vi "setConfiguration.vi"() -> (3 "TCPSettings out":refnum<class "TCPSettings.lvclass">)   [LabVIEW 2016]
uses:
  TCPSettings/TCPSettings.lvclass
  TCPSettings/TCPSettings.lvclass/TCPSettings.ctl
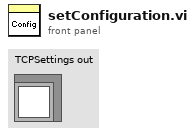
[diagram p1: front panel]
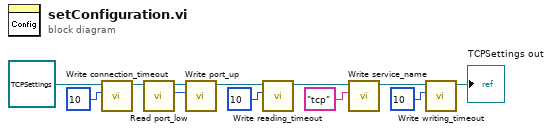
[diagram p0: block diagram]
diagram:
  n1 = call-dynamic "Write connection_timeout .vi"("connection_timeout"=10, "TCPSettings in"=refnum<class "TCPSettings.lvclass"> refnum ("TCPSettings.lvclass")) -> ("TCPSettings out"=w3:refnum<class "TCPSettings.lvclass">)  [unwired: 8 in, 1 out]
  n2 = call-dynamic "Read port_low.vi"("TCPSettings in"=w3) -> ("port_low"=w1:u16, "TCPSettings out"=w2:refnum<class "TCPSettings.lvclass">)  [unwired: 8 in, 1 out]
  n3 = call-dynamic "Write port_up.vi"("port_up"=w1, "TCPSettings in"=w2) -> ("TCPSettings out"=w11:refnum<class "TCPSettings.lvclass">)  [unwired: 8 in, 1 out]
  n4 = call-dynamic "Write reading_timeout.vi"("reading_timeout"=10, "TCPSettings in"=w11) -> ("TCPSettings out"=w10:refnum<class "TCPSettings.lvclass">)  [unwired: 8 in, 1 out]
  n5 = call "Write service_name.vi"("service_name"="tcp", "TCPSettings in"=w10) -> ("TCPSettings out"=w9:refnum<class "TCPSettings.lvclass">)  [unwired: 8 in, 1 out]
  n6 = call-dynamic "Write writing_timeout.vi"("writing_timeout"=10, "TCPSettings in"=w9) -> ("TCPSettings out"=→"TCPSettings out":refnum<class "TCPSettings.lvclass">)  [unwired: 8 in, 1 out]
